vi "Initialize.vi"(8 "error in (no error)":errorcluster, 10 "Configuration":T1, 11 "TCP_Streamer in":refnum<class "TCP_Streamer_Publisher.lvclass">) -> (0 "error out":errorcluster, 3 "TCP_Streamer out":refnum<class "TCP_Streamer_Publisher.lvclass">)   [LabVIEW 2021, in "TCP_Streamer_Publisher.lvclass"]
doc: "Create the listener and initialize the class.\n\n- IP address specifies on which network address to listen. Specifying an address is useful if you have more than one network card, such as two Ethernet cards, and want to listen only on the card with the specified address. If you do not specify a network address, this listens on all network addresses. \n\n- Port will set the listen port. If 0 then the OS will automatically choose an open port."
uses:
  TCP_Streamer_Publisher.lvclass
  Typedef/Configuration.ctl
  Typedef/State.ctl
  TCP_Streamer_Publisher.lvclass/TCP_Streamer_Publisher.ctl
  <vilib>/CIF Foundation/CIF Utilities/Networking/Networking_CIF_U.lvlib
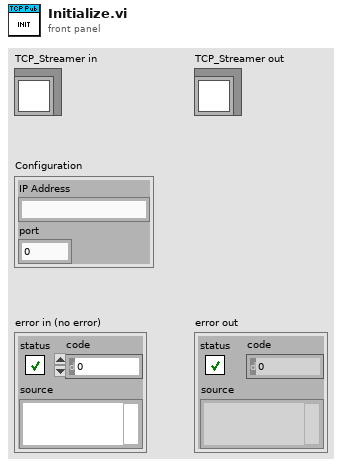
[diagram p1: front panel]
types:
  T1 = typedef "TCP_Streamer_Publisher.lvclass/Configuration.ctl" = cluster{"IP Address":string, "port":u16}
  T2 = typedef "TCP_Streamer_Publisher.lvclass/State.ctl" = enum16{"Stopped", "Listening", "Ready for Data", "Ready to Send", "Sending"}
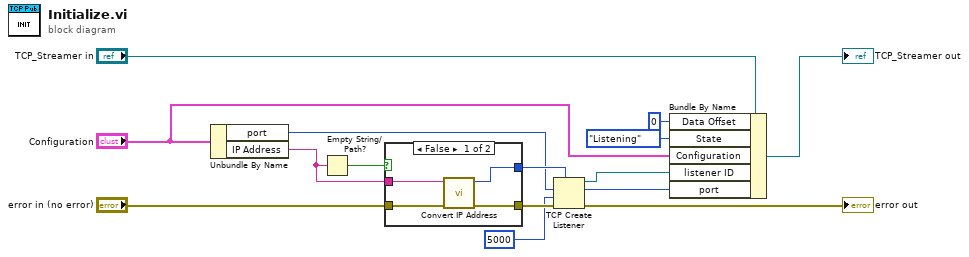
[diagram p0: block diagram]
diagram:
  n1 = Unbundle By Name("Configuration") -> ("port"=w9:u16, "IP Address"=w10:string)
  n2 = Empty String/Path?(string/path=w10) -> (empty?=w14:bool)
  n3 = case shown="False" w14 {
    tunnel: [w19 w20] -> w15
    tunnel: "error in (no error)" -> [w18 w20]
    tunnel: w10 -> [w17 _]
    tunnel: [w16 _] -> w13
    frame False {
      n4 = call <vilib>:"Convert IP Address.vi"("error in (no error)"=w18, "IP"=w17) -> ("error out"=w19:errorcluster, "net address"=w16:u32)  [unwired: 8 in]
    }
    frame True {
    }
  }
  n5 = TCP Create Listener(7:w13, 8:w15, 9:5000 ("timeout ms (25000)"), 10:w9) -> (0:→"error out":errorcluster, 2:w11:u16, 3:w3:refnum<k5>)  [unwired: 1 in]
  n6 = Bundle By Name(cluster="TCP_Streamer in", "Data Offset"=0, "State"=State."Listening", "Configuration"="Configuration", "listener ID"=w3, "port"=w11) -> (→"TCP_Streamer out":refnum<class "TCP_Streamer_Publisher.lvclass">)
